vi "calculate_power_in_chamber.vi"(9 "Aktuelle L/2 Position [°]":dbl, 10 "Eingestellte Polarisation [°]":dbl, 11 "Max. Leistung (vK) [mW]":dbl) -> (3 "Aktuelle Leistung (iK) [mW]":dbl)   [LabVIEW 2009]
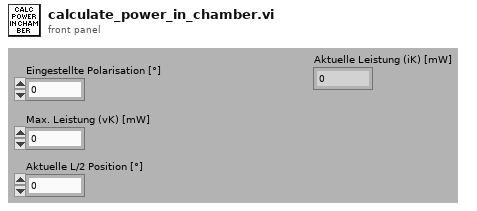
[diagram p1: front panel]
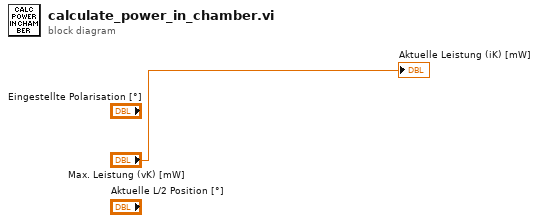
[diagram p0: block diagram]
diagram:
  "Aktuelle Leistung (iK) [mW]" <- "Max. Leistung (vK) [mW]"
